vi "Error code harness UI.vi"(10 "Color icon in":T1, 11 "BW icon in":T1) -> (0 "Error code out":i32, 2 "Color icon out":T1, 3 "BW icon out":T1)   [LabVIEW 2021, in "lv_icon.lvlib"]
uses:
  <vilib>/LabVIEW Icon API/lv_icon/lv_icon.lvlib
  <vilib>/picture/picture.llb/imagedata.ctl
panel:
  out "Previous state":picture
  in  "code":i32=1
  out "New state":picture
  in  "OK Button":bool
  # "Error code test harness"
  # "Code\n\n0 - Skips loading original icon editor.\n1 - Loads original icon editor with the changes from the custom one.\n 43 - Discard changes made to the editor (Cancel button)\nDefault - Loads original editor"
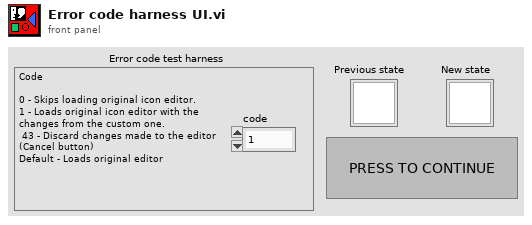
[diagram p1: front panel]
types:
  T1 = typedef "imagedata.ctl" = cluster{"image type":i32, "image depth":i32, "image":u8[], "mask":u8[], "colors":u32[], "Rectangle":cluster{"left":i16, "top":i16, "right":i16, "bottom":i16}}
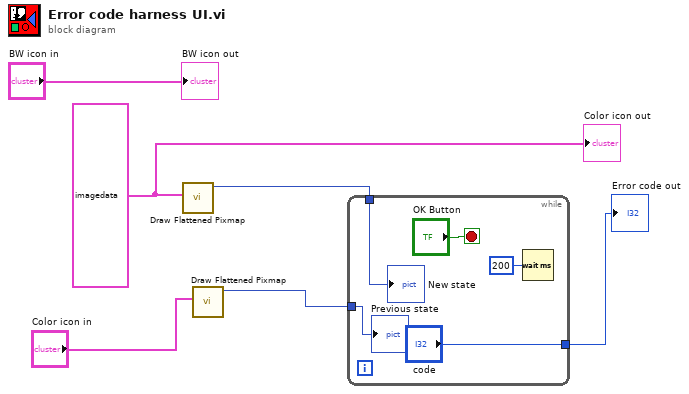
[diagram p0: block diagram]
diagram:
  w3 = T1 {"image type"=0, "image depth"=24, "image"=array[3072 elements], "mask"=[], "colors"=[], "Rectangle"={"left"=0, "top"=0, "right"=32, "bottom"=32}} ("image data")
  n1 = call <vilib>:"Draw Flattened Pixmap.vi"("image data"=w3) -> ("new picture"=w5:picture)  [unwired: 8 in]
  n2 = call <vilib>:"Draw Flattened Pixmap.vi"("image data"="Color icon in") -> ("new picture"=w2:picture)  [unwired: 8 in]
  n3 = while {
    tunnel: w5 -> [w9]
    tunnel: ["code"] -> w4
    tunnel: w2 -> [w7]
    stop <- "OK Button" stop-if-true
    n4 = Wait (ms)(milliseconds to wait=u32 200) -> ()  [unwired: 1 out]
    "New state" <- w9
    "Previous state" <- w7
  }
  "Error code out" <- w4
  "BW icon out" <- "BW icon in"
  "Color icon out" <- w3
